vi "CMN_FVAR_stop_coadd.vi"(8 "value in":bool, 9 "action":T1) -> (2 "value out":bool)   [LabVIEW 2016]
uses:
  CMN_FVAR_action.ctl
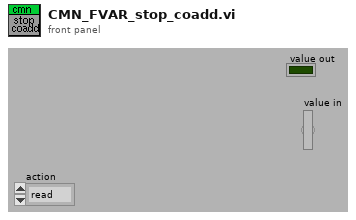
[diagram p1: front panel]
types:
  T1 = typedef "CMN_FVAR_action.ctl" = enum16{"read", "write"}
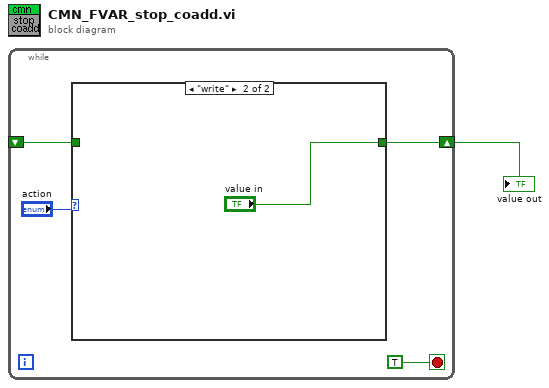
[diagram p0: block diagram]
diagram:
  n1 = while {
    shift-right: [w4] -> w1
    shift-left: _ -> [w3]
    stop <- TRUE stop-if-true
    n2 = case shown="\"write\"" "action" {
      tunnel: [w6 "value in"] -> w4
      tunnel: w3 -> [w6 _]
      frame "read", Default {
      }
      frame "write" {
      }
    }
  }
  "value out" <- w1
